vi "ThousandSons_FindCircle.vi"(8 "error in (no error)":errorcluster) -> (0 "error out":errorcluster)   [LabVIEW 2016]
uses:
  <vilib>/vision/NI_Vision_Development_Module.lvlib
panel:
  out "Circle Descriptor":T1
  out "Array":T2(array[cluster])
  in  "Color Plane":i32(ring)=1 items=["Red", "Green", "Blue", "Hue", "Saturation", "Luminance", "Value", "Intensity"]
  out "Image":T3(plugin-control)
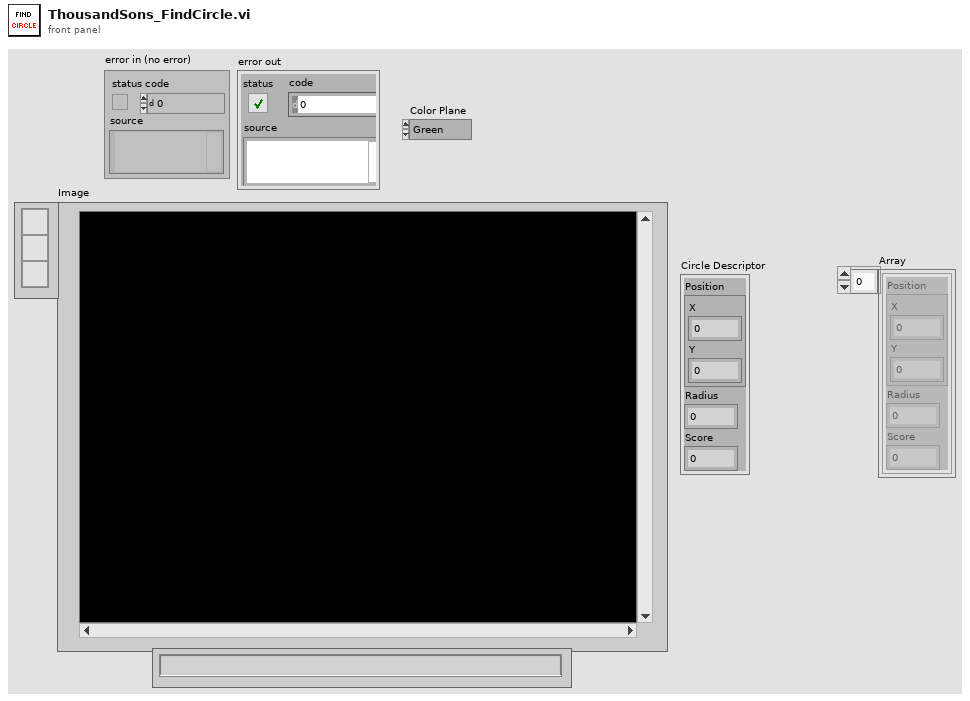
[diagram p1: front panel]
types:
  T1 = cluster{"Position":cluster{"X":sgl, "Y":sgl}, "Radius":dbl, "Score":dbl}
  T2 = cluster{"Position":cluster{"X":sgl, "Y":sgl}, "Radius":dbl, "Score":dbl}[]
  T3 = typedef "IMAQ Image.ctl" = refnum<image>
  T4 = typedef "IMAQ Circle" = cluster{"Center X":i32, "Center Y":i32, "Inner Radius":i32, "Outer Radius":i32, "Start Angle":dbl, "End Angle":dbl}
  T5 = typedef "ROI Descriptor" = cluster{"Global Rectangle":i32[], "Contours":cluster{"ID":enum32{"External", "Internal"}, "Type":u32, "Coordinates":i32[]}[]}
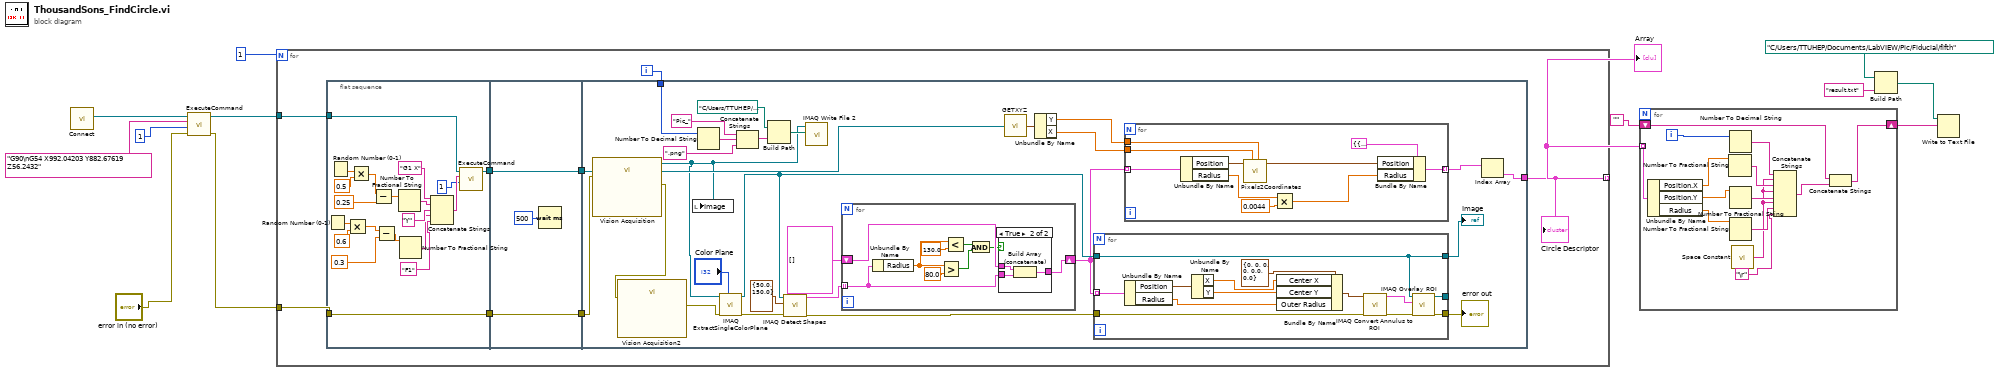
[diagram p0: block diagram]
diagram:
  n1 = call "Connect.vi"() -> ("controller"=w8:refnum<k24>)  [unwired: 10 in, 1 out]
  n2 = call "ExecuteCommand.vi"("error in (no error)"="error in (no error)", "taskId"=1, "Command Code"="G90\nG54 X992.04203 Y882.67619  Z56.2432", "controller in"=w8) -> ("error out"=w4:errorcluster, "controller out"=w7:refnum<k24>)  [unwired: 5 in, 1 out]
  n3 = for {
    N: 1 -> [_]
    tunnel: w4 -> [w17]
    tunnel: w7 -> [w16]
    tunnel: [w15] -> w6 mode=indexing
    i -> [w14]
    n4 = flat-sequence {
      tunnel: w17 -> [w41]
      tunnel: [w41] -> w21
      tunnel: w16 -> [w40]
      tunnel: [w39] -> w20
      tunnel: [w44] -> w19
      tunnel: w21 -> [w44]
      tunnel: w20 -> [w42]
      tunnel: [w42] -> w18
      tunnel: w19 -> [w46]
      tunnel: w18 -> [w56]
      tunnel: [w55] -> w15
      tunnel: w14 -> [w49]
      frame #0 {
        n5 = Random Number (0-1)() -> (number: 0 to 1=w33:dbl)
        n6 = Random Number (0-1)() -> (number: 0 to 1=w34:dbl)
        n7 = Multiply(x=w33, y=0.6) -> (x*y=w31:dbl)
        n8 = Multiply(x=w34, y=0.5) -> (x*y=w32:dbl)
        n9 = Subtract(x=w32, y=0.25) -> (x-y=w30:dbl)
        n10 = Subtract(x=w31, y=0.3) -> (x-y=w29:dbl)
        n11 = Number To Fractional String(number=w30) -> (F-format string=w27:string)  [unwired: 3 in]
        n12 = Number To Fractional String(number=w29) -> (F-format string=w28:string)  [unwired: 3 in]
        n13 = Concatenate Strings("G1 X", w27, "Y", w28, "F1") -> (w36:string)
        n14 = call "ExecuteCommand.vi"("taskId"=1, "Command Code"=w36, "controller in"=w40) -> ("controller out"=w39:refnum<k24>)  [unwired: 6 in, 2 out]
      }
      frame #1 {
        n15 = Wait (ms)(milliseconds to wait=u32 500) -> ()  [unwired: 1 out]
      }
      frame #2 {
        n16 = call "Vision Acquisition"("error in"=w46) -> ("Image Out"=w45:T3, "error out"=w47:errorcluster)  [unwired: 25 in]
        n17 = call "Vision Acquisition2"("error in"=w47) -> ("error out"=w57:errorcluster)  [unwired: 25 in, 1 out]
        n18 = local write "Image"(w45) -> ()
        n19 = Number To Decimal String(number=w49) -> (decimal integer string=w52:string)  [unwired: 1 in]
        n20 = call "IMAQ ExtractSingleColorPlane"("Color Plane"="Color Plane", "error in (no error)"=w57, "Image Src"=w45) -> ("error out"=w70:errorcluster, "Image Dst Out"=w67:T3)  [unwired: 7 in]
        n21 = Concatenate Strings("Pic_", w52, ".png") -> (w53:string)
        n22 = Build Path(base path=path "C:/Users/TTUHEP/Documents/LabVIEW/Pic/Fiducial/fifth", name or relative path=w53) -> (appended path=w54:path)
        n23 = call-poly "IMAQ Detect Shapes"("error in (no error)"=w70, "Circle Descriptor"=cluster{"Min Radius":dbl, "Max Radius":dbl} {"Min Radius"=50.0, "Max Radius"=150.0}, "Image"=w67) -> ("error out"=w68:errorcluster, "Circles"=w63:T2)  [unwired: 6 in, 1 out]
        n24 = call-poly "IMAQ Write File 2"("File Path"=w54, "Image"=w45) -> ()  [unwired: 8 in, 2 out]
        n25 = for {
          tunnel: w63 -> [w90] mode=indexing
          shift-right: [w87] -> w65
          shift-left: T2 [] ("Circle Descriptor") -> [w88]
          n26 = Unbundle By Name(w90) -> ("Radius"=w86:dbl)
          n27 = Greater?(x=w86, y=80.0) -> (0:w83:bool)
          n28 = Less?(x=w86, y=130.0) -> (x < y?=w84:bool)
          n29 = And(x=w84, y=w83) -> (x .and. y?=w82:bool)
          n30 = case shown="True" w82 {
            tunnel: w90 -> [_ w93]
            tunnel: w88 -> [w91 w94]
            tunnel: [w91 w92] -> w87
            frame False {
            }
            frame True {
              n31 = Build Array (concatenate)(w94, w93) -> (w92:T2)
            }
          }
        }
        n32 = call "GETXYZ.vi"(".NET Refnum in"=w56) -> ("XYZ"=w61:cluster{"X":dbl, "Y":dbl, "Z":dbl})
        n33 = Unbundle By Name(w61) -> ("Y"=w59:dbl, "X"=w60:dbl)
        n34 = for {
          tunnel: w65 -> [w107] mode=indexing
          tunnel: w67 -> [w97]
          tunnel: w68 -> [w99]
          tunnel: [w97] -> w64
          tunnel: [w96] -> w66
          tunnel: [w95] -> _
          n35 = Unbundle By Name(w107) -> ("Position"=w106:cluster{"X":sgl, "Y":sgl}, "Radius"=w101:dbl)
          n36 = Unbundle By Name(w106) -> ("X"=w103:sgl, "Y"=w102:sgl)
          n37 = Bundle By Name(cluster=T4 {"Center X"=0, "Center Y"=0, "Inner Radius"=0, "Outer Radius"=0, "Start Angle"=0.0, "End Angle"=0.0} ("Annulus"), "Center X"=w103, "Center Y"=w102, "Outer Radius"=w101) -> (w104:T4)
          n38 = call "IMAQ Convert Annulus to ROI"("error in (no error)"=w99, "Annulus"=w104) -> ("error out"=w98:errorcluster, "ROI Descriptor"=w100:T5)  [unwired: 7 in]
          n39 = call "IMAQ Overlay ROI"("error in (no error)"=w98, "ROI Descriptor"=w100, "Image"=w97) -> ("error out"=w96:errorcluster, "Image Out"=w95:T3)  [unwired: 7 in]
        }
        "Image" <- w64
        "error out" <- w66
        n40 = for {
          tunnel: w65 -> [w81] mode=indexing
          tunnel: [w74] -> w58 mode=indexing
          tunnel: w60 -> [w72]
          tunnel: w59 -> [w73]
          n41 = Unbundle By Name(w81) -> ("Position"=w76:cluster{"X":sgl, "Y":sgl}, "Radius"=w78:dbl)
          n42 = call "Pixels2Coordinates.vi"("Y"=w73, "X"=w72, "Location (Pixel)"=w76) -> ("output cluster"=w75:cluster{"X":sgl, "Y":sgl})  [unwired: 8 in]
          n43 = Multiply(x=w78, y=0.0044) -> (x*y=w79:dbl)
          n44 = Bundle By Name(cluster=T1 {"Position"={"X"=0.0, "Y"=0.0}, "Radius"=0.0, "Score"=0.0} ("Circle Descriptor"), "Position"=w75, "Radius"=w79) -> (w74:T1)
        }
        n45 = Index Array(array=w58) -> (element=w55:T1)  [unwired: 1 in]
      }
    }
    "Circle Descriptor" <- w15
  }
  "Array" <- w6
  n46 = for {
    tunnel: w6 -> [w121] mode=indexing
    shift-right: [w108] -> w12
    shift-left: "" -> [w109]
    i -> [w113]
    n47 = Unbundle By Name(w121) -> ("Position.X"=w120:sgl, "Position.Y"=w119:sgl, "Radius"=w118:dbl)
    n48 = Number To Fractional String(number=w120) -> (F-format string=w117:string)  [unwired: 3 in]
    n49 = Number To Decimal String(number=w113) -> (decimal integer string=w112:string)  [unwired: 1 in]
    n50 = Number To Fractional String(number=w119) -> (F-format string=w116:string)  [unwired: 3 in]
    n51 = Number To Fractional String(number=w118) -> (F-format string=w115:string)  [unwired: 3 in]
    n52 = call <vilib>:"Space Constant.vi"() -> ("String"=w114:string)
    n53 = Concatenate Strings(w112, w114, w117, w114, w116, w114, w115, "\r") -> (w110:string)
    n54 = Concatenate Strings(w109, w110) -> (w108:string)
  }
  n55 = Build Path(base path=path "C:/Users/TTUHEP/Documents/LabVIEW/Pic/Fiducial/fifth", name or relative path="result.txt") -> (appended path=w11:path)
  n56 = Write to Text File(file (use dialog)=w11, text=w12) -> ()  [unwired: 2 in, 3 out]
